vi "Day01-1.vi"() -> ()   [LabVIEW 2021]
panel:
  out "Counter":i64
  out "sum":i16
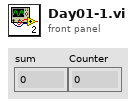
[diagram p1: front panel]
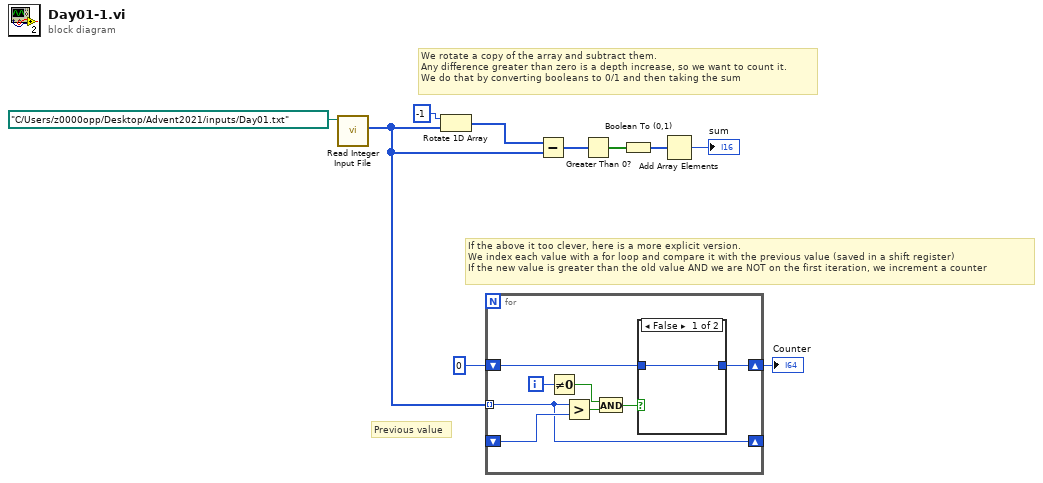
[diagram p0: block diagram]
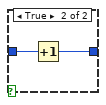
[diagram p2: hidden frame]
diagram:
  # "Previous value"
  # "If the above it too clever, here is a more explicit version.\nWe index each value with a for loop and compare it with the previous value (saved in a shift register)\nIf the new value is greater than the old value AND we are NOT on the first iteration, we increment a counter"
  # "We rotate a copy of the array and subtract them.\nAny difference greater than zero is a depth increase, so we want to count it.\nWe do that by converting booleans to 0/1 and then taking the sum"
  n1 = call "Read Integer Input File.vi"("file path (dialog if empty)"=path "C:/Users/z0000opp/Desktop/Advent2021/inputs/Day01.txt") -> ("input values"=w3:i64[])  [unwired: 10 in]
  n2 = Rotate 1D Array(1:w3, 2:-1 ("n")) -> (0:w9:i64[])
  n3 = for {
    tunnel: w3 -> [w15] mode=indexing
    shift-right: [w15] -> _
    shift-left: _ -> [w18]
    shift-right: [w16] -> w1
    shift-left: i64 0 -> [w17]
    i -> [w12]
    n4 = Not Equal To 0?(x=w12) -> (x != 0?=w11:bool)
    n5 = Greater?(x=w15, y=w18) -> (0:w13:bool)
    n6 = And(x=w11, y=w13) -> (x .and. y?=w14:bool)
    n7 = case shown="False" w14 {
      tunnel: w17 -> [w19 w21]
      tunnel: [w19 w20] -> w16
      frame False {
      }
      frame True {
        n8 = Increment(x=w21) -> (x+1=w20:i64)
      }
    }
  }
  "Counter" <- w1
  n9 = Subtract(x=w9, y=w3) -> (x-y=w7:i64[])
  n10 = Greater Than 0?(x=w7) -> (x > 0?=w6:bool[])
  n11 = Boolean To (0,1)(Boolean=w6) -> (0, 1=w5:i16[])
  n12 = Add Array Elements(numeric array=w5) -> (sum=→"sum":i16)
